vi "USBImageContinuousV1.2.vi"() -> ()   [LabVIEW 2019]
uses:
  <vilib>/Utility/file.llb/Write Delimited Spreadsheet (I64).vi
  Program Files (x86)/National Instruments/LabVIEW 2019/ATMCD32D.dll
panel:
  in  "Tab Control":T1(tab)
  out "Expected position on spectrometer (pixels):":dbl
  in  "Harmonic":dbl min=10.0 max=40.0
  out "l (nm)":dbl
  out "E (J)":dbl
  out "E (eV)":dbl
  out "Nearest Harmonic of 800nm":dbl
  out "Cursor Position (pixels)":dbl
  out "Distance to nearest harmonic of 800nm (pixels)":dbl
  in  "Grating:":u16(ring) items=["Shimadzu 30-006  "]
  in  "Laser:":u16(ring) items=["800nm  "]
  in  "Trigger":u32(ring) items=["Internal", "External"]
  out "Initialize":u32
  in  "Exposure Time (secs)":sgl format="%.2f"
  out "Calculated Exposure Value":sgl format="%.5f"
  out "Get Acquired Data":u32
  out "Start Acquisition":u32
  out "Detector X Pixels":i32
  out "Check Timings":u32
  out "Set Acquisition Mode":u32
  out "Set Readout Mode":u32
  out "Set Trigger Mode":u32
  out "Set Exposure Time":u32
  out "Get Detector":u32
  out "Detector Y Pixels":i32
  out "Shut Down":u32
  out "Set Gate Mode":u32
  out "Set Image":u32
  out "Raw Image From Camera":i32[][](graph)
  out "Vertical Binned Waveform Graph":i32[](graph)
  out "Get Status":u32
  in  "Stop":bool
  in  "?":bool
  out "Camera Status:":bool
  out "Last Image Saved:":string
  out "Wavelength Graph (nm)":cluster{"No prefix":dbl, i32}[](graph)
  out "Energy Graph (eV)":cluster{"eV":dbl, i32}[](graph)
  out "Harmonics Graph":cluster{"No prefix":dbl, i32}[](graph)
  out "Status":u32
  # "Status"
  # "Return values"
  # "Acquisition Mode: Single Scan\nReadout Mode: Full Resolution Image"
  # "XUV Spectrometer VI"
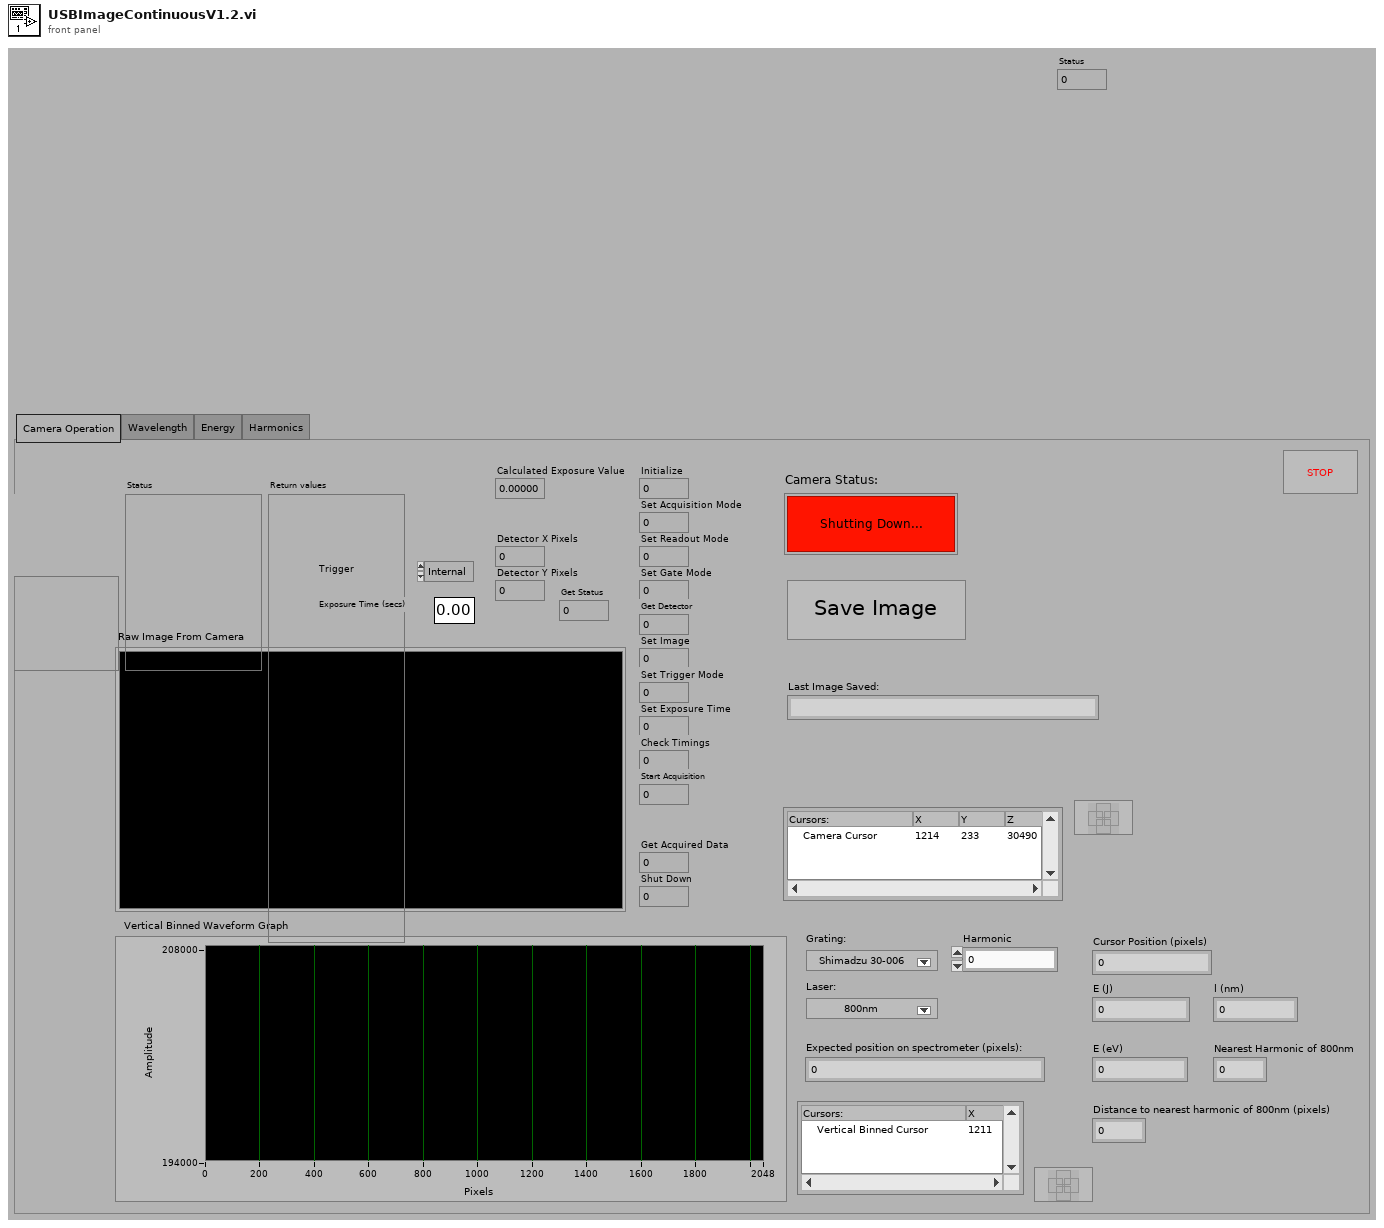
[diagram p1: front panel]
types:
  T1 = enum32{"Camera Operation", "Wavelength", "Energy", "Harmonics"}
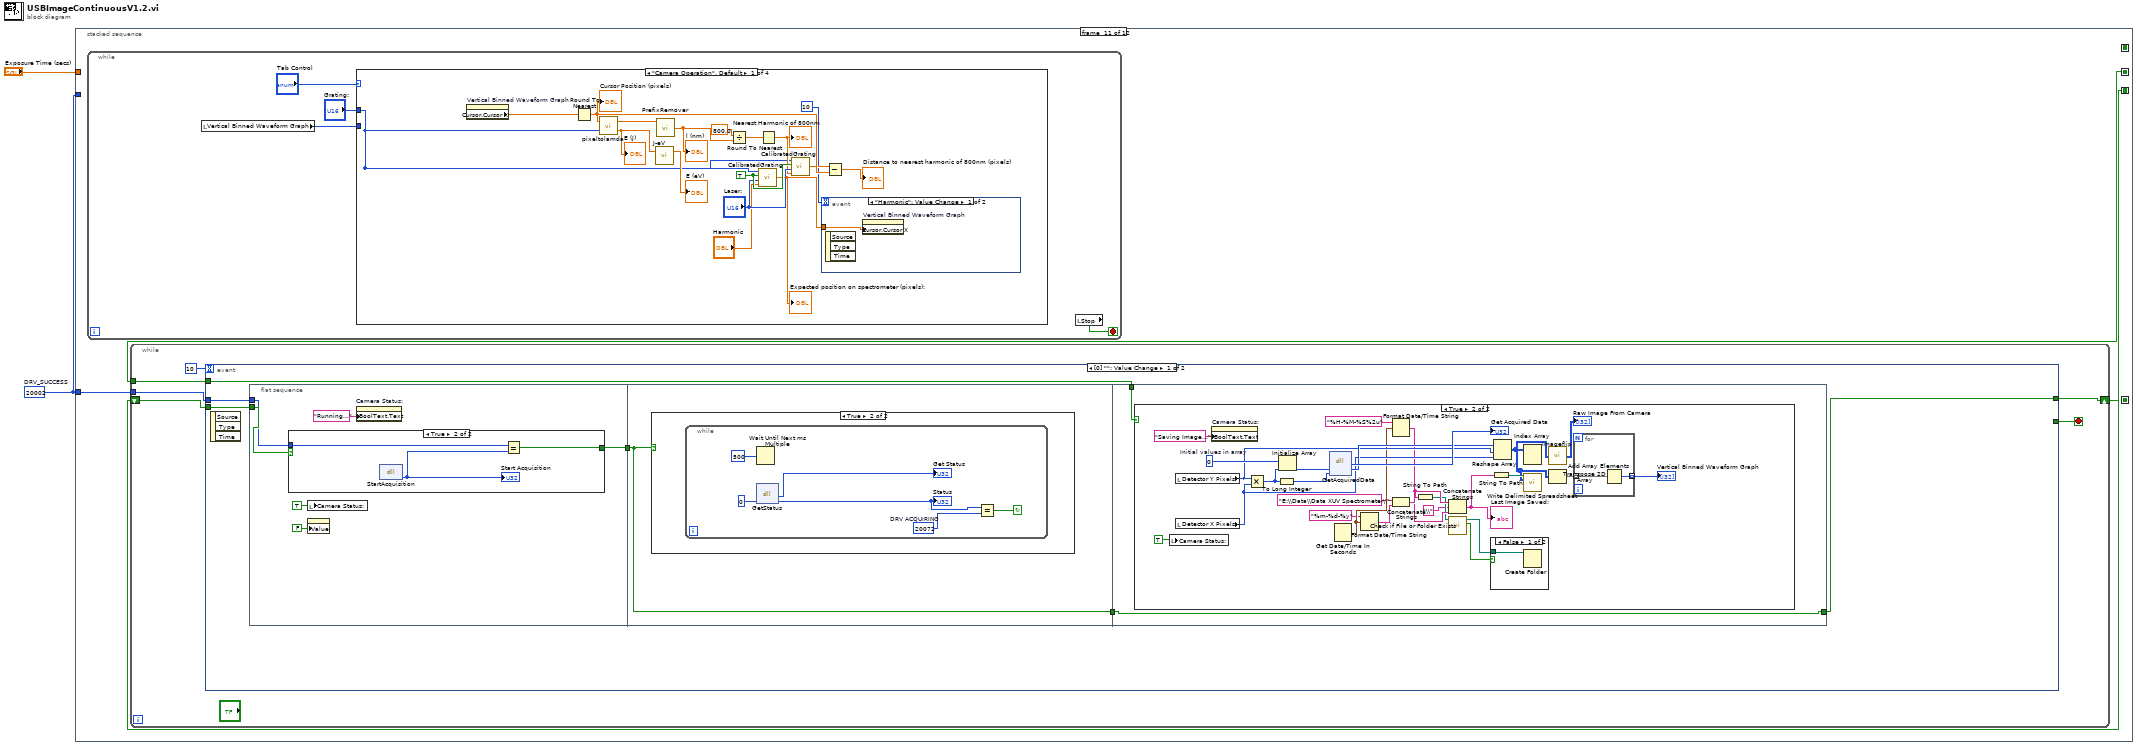
[diagram p0: block diagram]
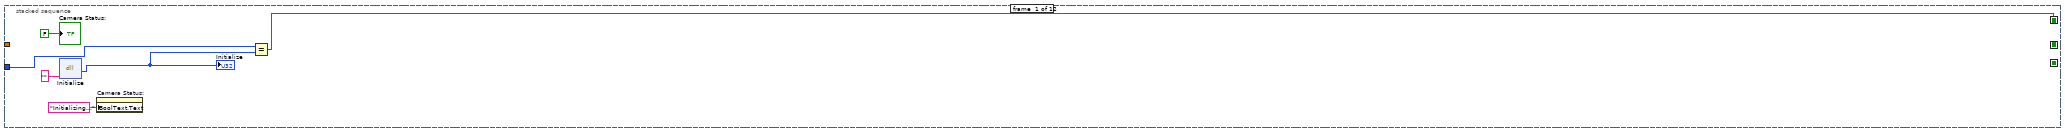
[diagram p2: hidden frame]
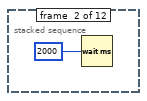
[diagram p3: hidden frame]
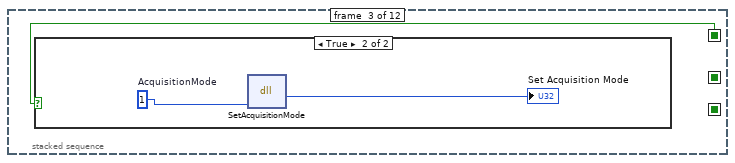
[diagram p4: hidden frame]
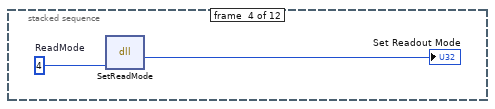
[diagram p6: hidden frame]
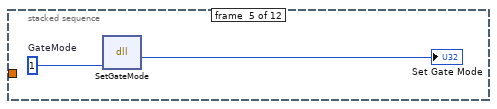
[diagram p7: hidden frame]
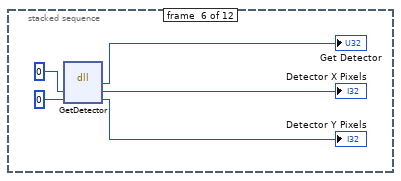
[diagram p8: hidden frame]
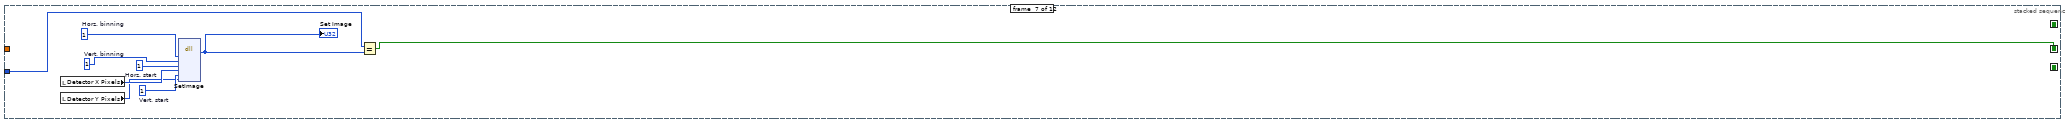
[diagram p9: hidden frame]
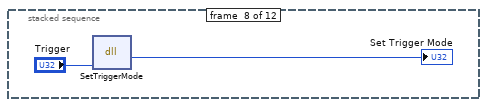
[diagram p10: hidden frame]
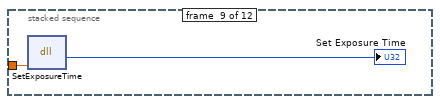
[diagram p11: hidden frame]
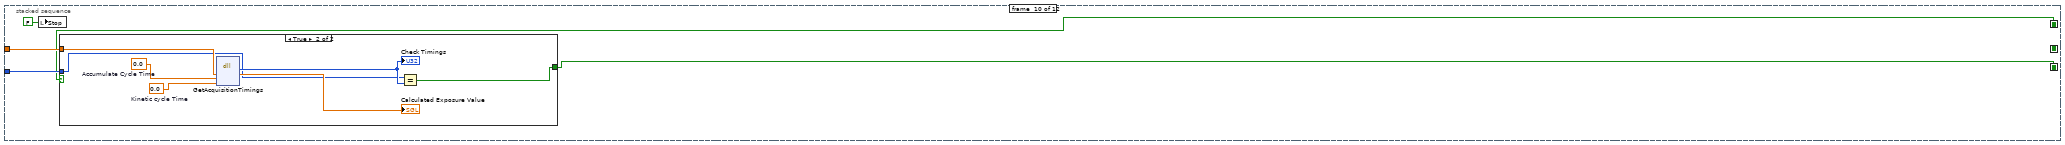
[diagram p12: hidden frame]
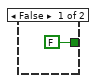
[diagram p13: hidden frame]
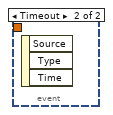
[diagram p14: hidden frame]
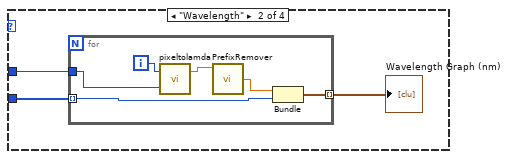
[diagram p15: hidden frame]
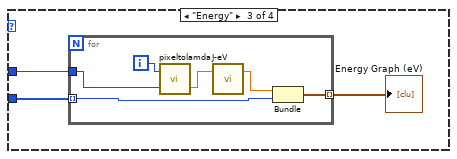
[diagram p16: hidden frame]
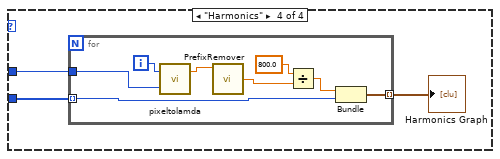
[diagram p17: hidden frame]
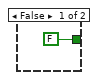
[diagram p18: hidden frame]
diagram:
  w1 = 20002  # DRV_SUCCESS
  n1 = stacked-sequence {
    seq-local: [w6 _ _ _ _ _ _ _ _ _ _ _] -> [_ _ w10 _ _ _ _ _ _ w36 _ w217]
    seq-local: [_ _ _ _ _ _ _ _ _ w37 _ _] -> [_ _ _ _ _ _ _ _ _ _ w51 _]
    seq-local: [_ _ _ _ _ _ _ _ _ _ w49 _] -> [_ _ _ _ _ _ _ _ _ _ _ _]
    seq-local: [_ _ _ _ _ _ w22 _ _ _ _ _] -> [_ _ _ _ _ _ _ _ _ _ w48 _]
    tunnel: "Exposure Time (secs)" -> [_ _ _ _ _ _ _ _ w34 w39 _ _]
    tunnel: w1 -> [w7 _ _ _ _ _ w24 _ _ w38 _ _]
    tunnel: w1 -> [_ _ _ _ _ _ _ _ _ _ w50 _]
    frame #0 {
      n2 = dll-call lib="C:/Program Files (x86)/National Instruments/LabVIEW 2019/atmcd32d.dll" fn="Initialize" label="Call Library Function Initialize"("") -> (w8:u32)  [unwired: 4 in, 2 out]
      "Initialize" <- w8
      n3 = property on="Camera Status:" class="Bool (strict)"("BoolText.Text"="Initializing..." ("String")) -> ()  [unwired: 2 in, 2 out]
      n4 = Equal?(x=w7, y=w8) -> (x = y?=w6:bool)
      "Camera Status:" <- FALSE ("Camera Status:")
    }
    frame #1 {
      n5 = Wait (ms)(milliseconds to wait=u32 2000) -> ()  [unwired: 1 out]
    }
    frame #2 {
      n6 = case shown="True" w10 {
        frame False {
        }
        frame True {
          w12 = u16 1  # AcquisitionMode
          n7 = dll-call lib="C:/Program Files (x86)/National Instruments/LabVIEW 2019/atmcd32d.dll" fn="SetAcquisitionMode" label="Call Library Function SetAcquisitionMode"(w12) -> (→"Set Acquisition Mode":u32)  [unwired: 4 in, 2 out]
        }
      }
    }
    frame #3 {
      w14 = u16 4  # ReadMode
      n8 = dll-call lib="C:/Program Files (x86)/National Instruments/LabVIEW 2019/atmcd32d.dll" fn="SetReadMode" label="Call Library Function SetReadMode"(w14) -> (→"Set Readout Mode":u32)  [unwired: 4 in, 2 out]
    }
    frame #4 {
      w16 = u16 1  # GateMode
      n9 = dll-call lib="C:/Program Files (x86)/National Instruments/LabVIEW 2019/atmcd32d.dll" fn="SetGateMode" label="Call Library Function SetGateMode"(w16) -> (→"Set Gate Mode":u32)  [unwired: 4 in, 2 out]
    }
    frame #5 {
      n10 = dll-call lib="C:/Program Files (x86)/National Instruments/LabVIEW 2019/atmcd32d.dll" fn="GetDetector" label="Call Library FunctionGetDetector"(i16 0, i16 0) -> (→"Get Detector":u32, →"Detector X Pixels":i32, →"Detector Y Pixels":i32)  [unwired: 3 in, 2 out]
    }
    frame #6 {
      w27 = u16 1  # Vert. start
      w28 = u16 1  # Horz. start
      w29 = u16 1  # Vert. binning
      w30 = u16 1  # Horz. binning
      n11 = local read "Detector X Pixels"() -> (w26:i32)
      n12 = local read "Detector Y Pixels"() -> (w25:i32)
      n13 = dll-call lib="C:/Program Files (x86)/National Instruments/LabVIEW 2019/atmcd32d.dll" fn="SetImage" label="Call Library Function SetImage"(w30, w29, w28, w26, w27, w25) -> (w23:u32)  [unwired: 9 in, 2 out]
      "Set Image" <- w23
      n14 = Equal?(x=w24, y=w23) -> (x = y?=w22:bool)
    }
    frame #7 {
      n15 = dll-call lib="C:/Program Files (x86)/National Instruments/LabVIEW 2019/atmcd32d.dll" fn="SetTriggerMode" label="Call Library Function SetTrigger Mode"("Trigger") -> (→"Set Trigger Mode":u32)  [unwired: 4 in, 2 out]
    }
    frame #8 {
      n16 = dll-call lib="C:/Program Files (x86)/National Instruments/LabVIEW 2019/atmcd32d.dll" fn="SetExposureTime" label="Call Library FunctionSet Exposure Time"(w34) -> (→"Set Exposure Time":u32)  [unwired: 4 in, 2 out]
    }
    frame #9 {
      n17 = local write "Stop"(FALSE ("Stop")) -> ()
      n18 = case shown="True" w36 {
        tunnel: w39 -> [_ w44]
        tunnel: w38 -> [_ w41]
        tunnel: [FALSE w43] -> w37
        frame False {
        }
        frame True {
          w46 = sgl 0.0  # Accumulate Cycle Time
          w47 = sgl 0.0  # Kinetic cycle Time
          n19 = dll-call lib="C:/Program Files (x86)/National Instruments/LabVIEW 2019/atmcd32d.dll" fn="GetAcquisitionTimings" label="Call Library Function Check Timings"(w44, w46, w47) -> (w42:u32, →"Calculated Exposure Value":sgl)  [unwired: 5 in, 2 out]
          "Check Timings" <- w42
          n20 = Equal?(x=w41, y=w42) -> (x = y?=w43:bool)
        }
      }
    }
    frame #10 {
      n21 = while {
        stop <- w52 stop-if-true
        n22 = local read "Vertical Binned Waveform Graph"() -> (w54:i32[])
        n23 = case shown="\"Camera Operation\", Default" "Tab Control" {
          tunnel: w54 -> [_ w76 w85 w94]
          tunnel: "Grating:" -> [w56 w75 w84 w93]
          frame "Camera Operation", Default {
            w72 = TRUE
            n24 = property on="Vertical Binned Waveform Graph" class="WFGraph (strict)"() -> ("Cursor.Cursor X"=w69:dbl)  [unwired: 2 in, 2 out]
            n25 = Round To Nearest(number=w69) -> (nearest integer value=w62:dbl)
            "Cursor Position (pixels)" <- w62
            n26 = call "pixeltolamda.vi"("Grating:"=w56, "Pixel Postion"=w62) -> ("E (J)"=w64:dbl, "lamda (m)"=w70:dbl)
            "E (J)" <- w64
            n27 = call "J-eV.vi"("J"=w64) -> ("eV"=→"E (eV)":dbl)  [unwired: 1 in, 1 out]
            n28 = call "PrefixRemover.vi"("Nano"=w70) -> ("No prefix"=w65:dbl)  [unwired: 3 in]
            "l (nm)" <- w65
            n29 = Divide(x=800.0, y=w65) -> (x/y=w67:dbl)
            n30 = call "CalibratedGrating.vi"("Harmonic"="Harmonic", "Laser:"="Laser:", "Subvi?"=w72, "Grating:"=w56) -> ("Position on spectrometer (pixels):"=w58:dbl)
            "Expected position on spectrometer (pixels):" <- w58
            n31 = Round To Nearest(number=w67) -> (nearest integer value=w61:dbl)
            "Nearest Harmonic of 800nm" <- w61
            n32 = call "CalibratedGrating.vi"("Harmonic"=w61, "Laser:"="Laser:", "Subvi?"=w72, "Grating:"=w56) -> ("Position on spectrometer (pixels):"=w60:dbl)
            n33 = event shown="[0] \"Harmonic\": Value Change" {
              selector: _ -> [_ _]
              dyn-events: _ -> [_ _]
              timeout: 10 -> [_ _]
              tunnel: w58 -> [w73 _]
              event "Harmonic": Value Change {
                n34 = event-data() -> ()  [unwired: 1 in, 3 out]
                n35 = property on="Vertical Binned Waveform Graph" class="WFGraph (strict)"("Cursor.Cursor X"=w73) -> ()  [unwired: 2 in, 2 out]
              }
              event Timeout {
                n36 = event-data() -> ()  [unwired: 1 in, 3 out]
              }
            }
            n37 = Subtract(x=w60, y=w62) -> (x-y=→"Distance to nearest harmonic of 800nm (pixels)":dbl)
          }
          frame "Wavelength" {
            n38 = for {
              tunnel: w76 -> [w78] mode=indexing
              tunnel: w75 -> [w80]
              tunnel: [w77] -> w74 mode=indexing
              i -> [w79]
              n39 = call "pixeltolamda.vi"("Grating:"=w80, "Pixel Postion"=w79) -> ("lamda (m)"=w81:dbl)  [unwired: 1 out]
              n40 = call "PrefixRemover.vi"("Nano"=w81) -> ("No prefix"=w82:dbl)  [unwired: 3 in]
              n41 = Bundle("No prefix"=w82, w78) -> (w77:cluster{"No prefix":dbl, i32})  [unwired: 1 in]
            }
            "Wavelength Graph (nm)" <- w74
          }
          frame "Energy" {
            n42 = for {
              tunnel: w85 -> [w87] mode=indexing
              tunnel: w84 -> [w90]
              tunnel: [w86] -> w83 mode=indexing
              i -> [w91]
              n43 = call "pixeltolamda.vi"("Grating:"=w90, "Pixel Postion"=w91) -> ("E (J)"=w89:dbl)  [unwired: 1 out]
              n44 = call "J-eV.vi"("J"=w89) -> ("eV"=w88:dbl)  [unwired: 1 in, 1 out]
              n45 = Bundle("eV"=w88, w87) -> (w86:cluster{"eV":dbl, i32})  [unwired: 1 in]
            }
            "Energy Graph (eV)" <- w83
          }
          frame "Harmonics" {
            n46 = for {
              tunnel: w94 -> [w99] mode=indexing
              tunnel: w93 -> [w101]
              tunnel: [w98] -> w92 mode=indexing
              i -> [w100]
              n47 = call "pixeltolamda.vi"("Grating:"=w101, "Pixel Postion"=w100) -> ("lamda (m)"=w102:dbl)  [unwired: 1 out]
              n48 = call "PrefixRemover.vi"("Nano"=w102) -> ("No prefix"=w96:dbl)  [unwired: 3 in]
              n49 = Divide(x=800.0, y=w96) -> (x/y=w95:dbl)
              n50 = Bundle(w95, w99) -> (w98:cluster{dbl, i32})  [unwired: 1 in]
            }
            "Harmonics Graph" <- w92
          }
        }
        n51 = local read "Stop"() -> (w52:bool)
      }
      n52 = while {
        tunnel: w50 -> [w107]
        tunnel: w48 -> [w105]
        shift-right: [w106] -> w49
        shift-left: w51 -> [w108]
        stop <- w103 stop-if-true
        n53 = event shown="[0] \"\": Value Change" {
          selector: _ -> [_ _]
          dyn-events: _ -> [_ _]
          timeout: 10 -> [_ _]
          tunnel: w108 -> [w112 w169]
          tunnel: w107 -> [w111 w168]
          tunnel: [w110 w167] -> w106
          tunnel: w105 -> [w109 w166]
          tunnel: [_ w165] -> w103
          event Value Change {
            n54 = event-data() -> ()  [unwired: 1 in, 3 out]
            n55 = flat-sequence {
              tunnel: w112 -> [w120]
              tunnel: w111 -> [w119]
              tunnel: [w118] -> w114
              tunnel: w114 -> [w125]
              tunnel: [w125] -> w113
              tunnel: [w133] -> w110
              tunnel: w113 -> [w133]
              tunnel: w109 -> [w132]
              frame #0 {
                n56 = case shown="True" w120 {
                  tunnel: [FALSE w123] -> w118
                  tunnel: w119 -> [_ w122]
                  frame False {
                  }
                  frame True {
                    n57 = dll-call lib="C:/Program Files (x86)/National Instruments/LabVIEW 2019/atmcd32d.dll" fn="StartAcquisition" label="Call Library Function start acquisition"() -> (w124:u32)  [unwired: 3 in, 2 out]
                    "Start Acquisition" <- w124
                    n58 = Equal?(x=w122, y=w124) -> (x = y?=w123:bool)
                  }
                }
                n59 = local write "Camera Status:"(TRUE ("Camera Status:")) -> ()
                n60 = property class="Bool (strict)"("Value"=FALSE ("Take image")) -> ()  [unwired: 2 in, 2 out]
                n61 = property on="Camera Status:" class="Bool (strict)"("BoolText.Text"="Running..." ("Boolean Text.Text")) -> ()  [unwired: 2 in, 2 out]
              }
              frame #1 {
                n62 = case shown="True" w125 {
                  frame False {
                  }
                  frame True {
                    n63 = while {
                      stop <- w129 continue-if-true
                      w128 = u16 20072  # DRV ACQUIRING
                      n64 = Wait Until Next ms Multiple(millisecond multiple=u32 500) -> ()  [unwired: 1 out]
                      n65 = dll-call lib="C:/Program Files (x86)/National Instruments/LabVIEW 2019/atmcd32d.dll" fn="GetStatus" label="Call Library Function GetAcquisitionStatus"(u16 0) -> (→"Get Status":u32, w127:u32)  [unwired: 3 in, 2 out]
                      "Status" <- w127
                      n66 = Equal?(x=w127, y=w128) -> (x = y?=w129:bool)
                    }
                  }
                }
              }
              frame #2 {
                n67 = case shown="True" w132 {
                  frame False {
                  }
                  frame True {
                    w160 = 0  # Initial values in array
                    n68 = local write "Camera Status:"(TRUE ("Camera Status:")) -> ()
                    n69 = local read "Detector Y Pixels"() -> (w154:i32)
                    n70 = local read "Detector X Pixels"() -> (w153:i32)
                    n71 = property on="Camera Status:" class="Bool (strict)"("BoolText.Text"="Saving Image..." ("Boolean Text.Text")) -> ()  [unwired: 2 in, 2 out]
                    n72 = Multiply(x=w154, y=w153) -> (x*y=w156:i32)
                    n73 = To Long Integer(number=w156) -> (32bit integer=w157:i32)
                    n74 = Initialize Array "Initialize Array"(w160, w156) -> (w158:i32[])
                    n75 = dll-call lib="C:/Program Files (x86)/National Instruments/LabVIEW 2019/atmcd32d.dll" fn="GetAcquiredData" label="Call Library Function Get Acquired data"(w158, w157) -> (→"Get Acquired Data":u32, w155:i32[])  [unwired: 4 in, 2 out]
                    n76 = Get Date/Time In Seconds() -> (seconds since 1Jan1904=w150:timestamp)
                    n77 = Format Date/Time String(time format string (%c)="%m-%d-%y", seconds (now)=w150) -> (date/time string=w148:string)  [unwired: 1 in]
                    n78 = Format Date/Time String(time format string (%c)="%H-%M-%S%2u", seconds (now)=w150) -> (date/time string=w149:string)  [unwired: 1 in]
                    n79 = Concatenate Strings("E:\\Data\\Data XUV Spectrometer\\" ("string"), w148) -> (w151:string)
                    n80 = String To Path(string=w151) -> (path=w147:path)
                    n81 = Concatenate Strings(w151, "\\" ("string"), w149) -> (w152:string)
                    "Last Image Saved:" <- w152
                    n82 = call <vilib>:"Check if File or Folder Exists.vi"("path"=w147) -> ("file or folder exists?"=w145:bool, "dup path"=w146:path)  [unwired: 8 in, 1 out]
                    n83 = case shown="False" w145 {
                      tunnel: w146 -> [w163 _]
                      frame False {
                        n84 = Create Folder(path (use dialog)=w163) -> ()  [unwired: 2 in, 3 out]
                      }
                      frame True {
                      }
                    }
                    n85 = String To Path(string=w152) -> (path=w140:path)
                    n86 = Reshape Array(w155, w154, w153) -> (w135:i32[][])
                    n87 = Index Array(array=w135) -> ()  [unwired: 2 in, 1 out]
                    n88 = call-poly <vilib>:"Write Delimited Spreadsheet.vi"("file path (dialog if empty)"=w140, "2D data"=w135) -> ()  [unwired: 12 in, 2 out]
                    n89 = call "Imageflip.vi"("2D array"=w135) -> ("transposed array"=→"Raw Image From Camera":i32[][])
                    n90 = Transpose 2D Array(2D array=w135) -> (transposed array=w139:i32[][])
                    n91 = for {
                      tunnel: w139 -> [w162] mode=indexing
                      tunnel: [w161] -> w138 mode=indexing
                      n92 = Add Array Elements(numeric array=w162) -> (sum=w161:i32)
                    }
                    "Vertical Binned Waveform Graph" <- w138
                  }
                }
              }
            }
          }
          event Timeout {
            n93 = event-data() -> ()  [unwired: 1 in, 3 out]
            n94 = flat-sequence {
              tunnel: w169 -> [w176]
              tunnel: w168 -> [w175]
              tunnel: [w174] -> w171
              tunnel: w171 -> [w181]
              tunnel: [w181] -> w170
              tunnel: w170 -> [w188]
              tunnel: w166 -> [w189]
              tunnel: [w188] -> w164
              tunnel: ["Stop"] -> w165
              tunnel: [w214] -> w167
              tunnel: w164 -> [w214]
              frame #0 {
                n95 = case shown="True" w176 {
                  tunnel: [FALSE w180] -> w174
                  tunnel: w175 -> [_ w179]
                  frame False {
                  }
                  frame True {
                    n96 = dll-call lib="C:/Program Files (x86)/National Instruments/LabVIEW 2019/atmcd32d.dll" fn="StartAcquisition" label="Call Library Function start acquisition"() -> (w178:u32)  [unwired: 3 in, 2 out]
                    n97 = local write "Start Acquisition"(w178) -> ()
                    n98 = Equal?(x=w179, y=w178) -> (x = y?=w180:bool)
                  }
                }
                n99 = local write "Camera Status:"(TRUE ("Camera Status:")) -> ()
                n100 = property on="Camera Status:" class="Bool (strict)"("BoolText.Text"="Running..." ("Boolean Text.Text")) -> ()  [unwired: 2 in, 2 out]
              }
              frame #1 {
                n101 = case shown="True" w181 {
                  frame False {
                  }
                  frame True {
                    n102 = while {
                      stop <- w185 continue-if-true
                      w184 = u16 20072  # DRV ACQUIRING
                      n103 = Wait Until Next ms Multiple(millisecond multiple=u32 500) -> ()  [unwired: 1 out]
                      n104 = dll-call lib="C:/Program Files (x86)/National Instruments/LabVIEW 2019/atmcd32d.dll" fn="GetStatus" label="Call Library Function GetAcquisitionStatus"(u16 0) -> (w183:u32, w182:u32)  [unwired: 3 in, 2 out]
                      n105 = local write "Status"(w182) -> ()
                      n106 = local write "Get Status"(w183) -> ()
                      n107 = Equal?(x=w182, y=w184) -> (x = y?=w185:bool)
                    }
                  }
                }
              }
              frame #2 {
                n108 = case shown="True" w189 {
                  frame False {
                  }
                  frame True {
                    w204 = 0  # Initial values in array
                    n109 = local read "Detector Y Pixels"() -> (w199:i32)
                    n110 = local read "Detector X Pixels"() -> (w198:i32)
                    n111 = Multiply(x=w199, y=w198) -> (x*y=w201:i32)
                    n112 = Initialize Array "Initialize Array"(w204, w201) -> (w203:i32[])
                    n113 = To Long Integer(number=w201) -> (32bit integer=w202:i32)
                    n114 = dll-call lib="C:/Program Files (x86)/National Instruments/LabVIEW 2019/atmcd32d.dll" fn="GetAcquiredData" label="Call Library Function Get Acquired data"(w203, w202) -> (w196:u32, w200:i32[])  [unwired: 4 in, 2 out]
                    n115 = local write "Get Acquired Data"(w196) -> ()
                    n116 = Reshape Array(w200, w199, w198) -> (w190:i32[][])
                    n117 = Index Array(array=w190) -> ()  [unwired: 2 in, 1 out]
                    n118 = Array Max & Min(array=w190) -> (max value=w194:i32)  [unwired: 3 out]
                    n119 = Transpose 2D Array(2D array=w190) -> (transposed array=w197:i32[][])
                    n120 = call "Imageflip.vi"("2D array"=w190) -> ("transposed array"=w191:i32[][])
                    n121 = local write "Raw Image From Camera"(w191) -> ()
                    n122 = for {
                      tunnel: w197 -> [w212] mode=indexing
                      tunnel: [w211] -> w195 mode=indexing
                      n123 = Add Array Elements(numeric array=w212) -> (sum=w211:i32)
                    }
                    n124 = Greater?(x=w194, y=64900) -> (0:w192:bool)
                    n125 = case shown="True" w192 {
                      frame False {
                      }
                      frame True {
                        n126 = local write "Camera Status:"(FALSE ("Camera Status:")) -> ()
                        n127 = property on="Camera Status:" class="Bool (strict)"("BoolText.Text"="Saturated!" ("Boolean Text.Text")) -> ()  [unwired: 2 in, 2 out]
                        n128 = Two Button Dialog(message="Camera is saturating! Reduce photon flux!", 1:"I've fixed it, and I want to continue" ("message"), 2:"Shut Down Camera" ("T button name (\"OK\")")) -> (T button?=w206:bool)
                        n129 = local write "Stop"(w206) -> ()
                      }
                    }
                    n130 = local write "Vertical Binned Waveform Graph"(w195) -> ()
                  }
                }
              }
              frame #3 {
              }
            }
          }
        }
      }
    }
    frame #11 {
      n131 = local write "Camera Status:"(FALSE ("Camera Status:")) -> ()
      n132 = property on="Camera Status:" class="Bool (strict)"("BoolText.Text"="Shutting Down..." ("Boolean Text.Text")) -> ()  [unwired: 2 in, 2 out]
      n133 = case shown="True" w217 {
        frame False {
        }
        frame True {
          n134 = dll-call lib="C:/Program Files (x86)/National Instruments/LabVIEW 2019/atmcd32d.dll" fn="ShutDown" label="Call Library Function Shutdown"() -> (→"Shut Down":u32)  [unwired: 3 in, 2 out]
        }
      }
    }
  }
